vi "time_duration.vi"(8 "error in (no error)":errorcluster, 9 "out time":string[](array[string]), 10 "in time":string[](array[string]), 11 "Numeric":i32) -> (0 "error out":errorcluster, 1 "x+y 2":i32[](array[numeric]), 2 "time in second":dbl[](array[numeric]), 3 "x+y":i32[](array[numeric]))   [LabVIEW 2017]
panel:
  out "x+y 3":i32[](array[numeric])
  out "number 2":i32[](array[numeric])
  out "number":i32[](array[numeric])
  in  "Array 4":string[](array[string])
  out "Array 3":i32[](array[numeric])
  out "Array 2":i32[](array[numeric])
  out "Array":i32[](array[numeric])
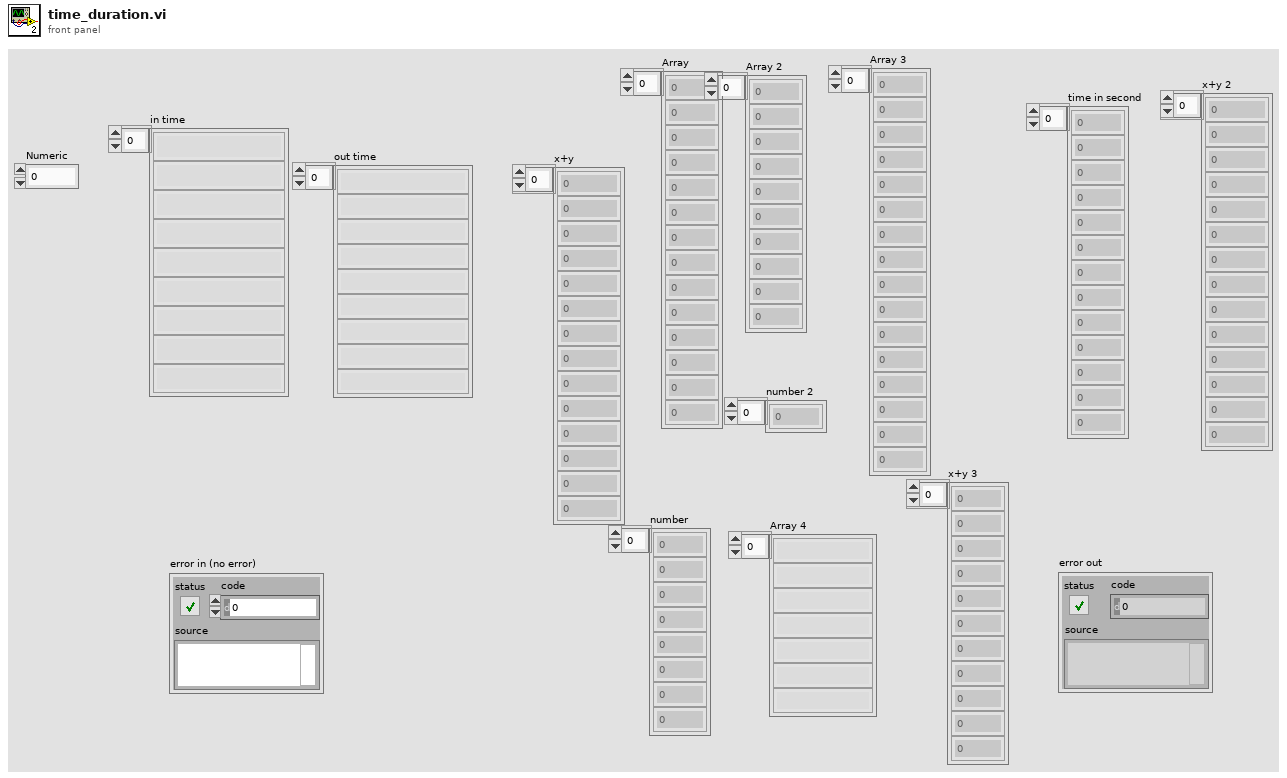
[diagram p1: front panel]
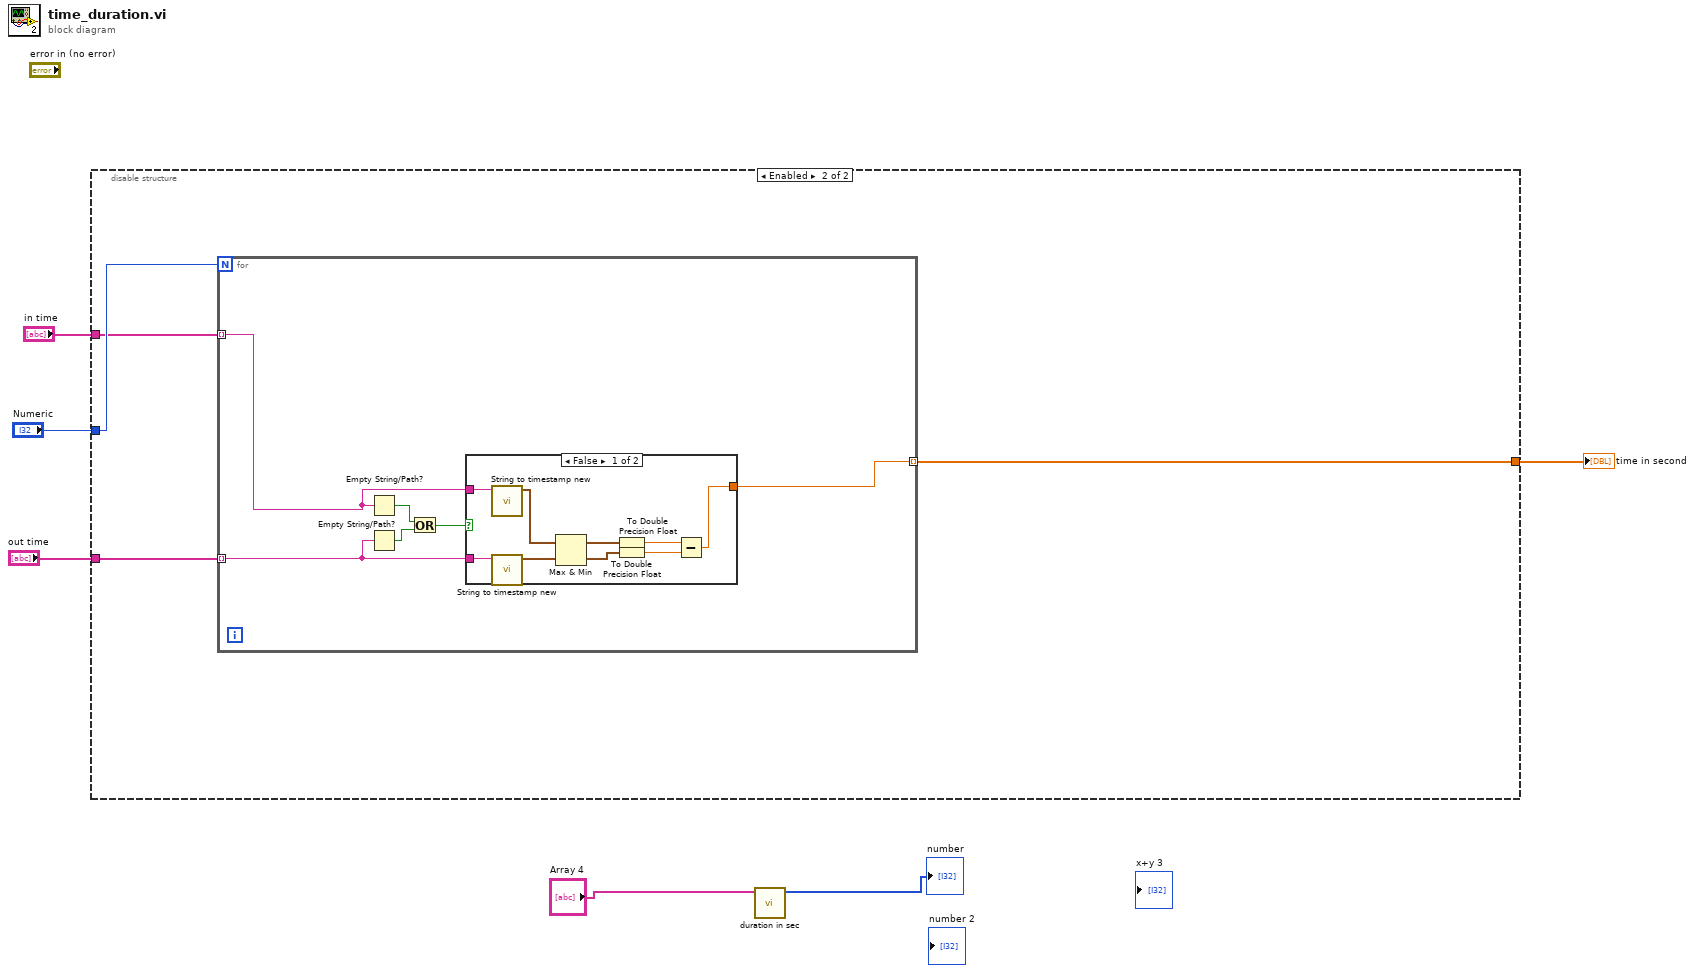
[diagram p0: block diagram]
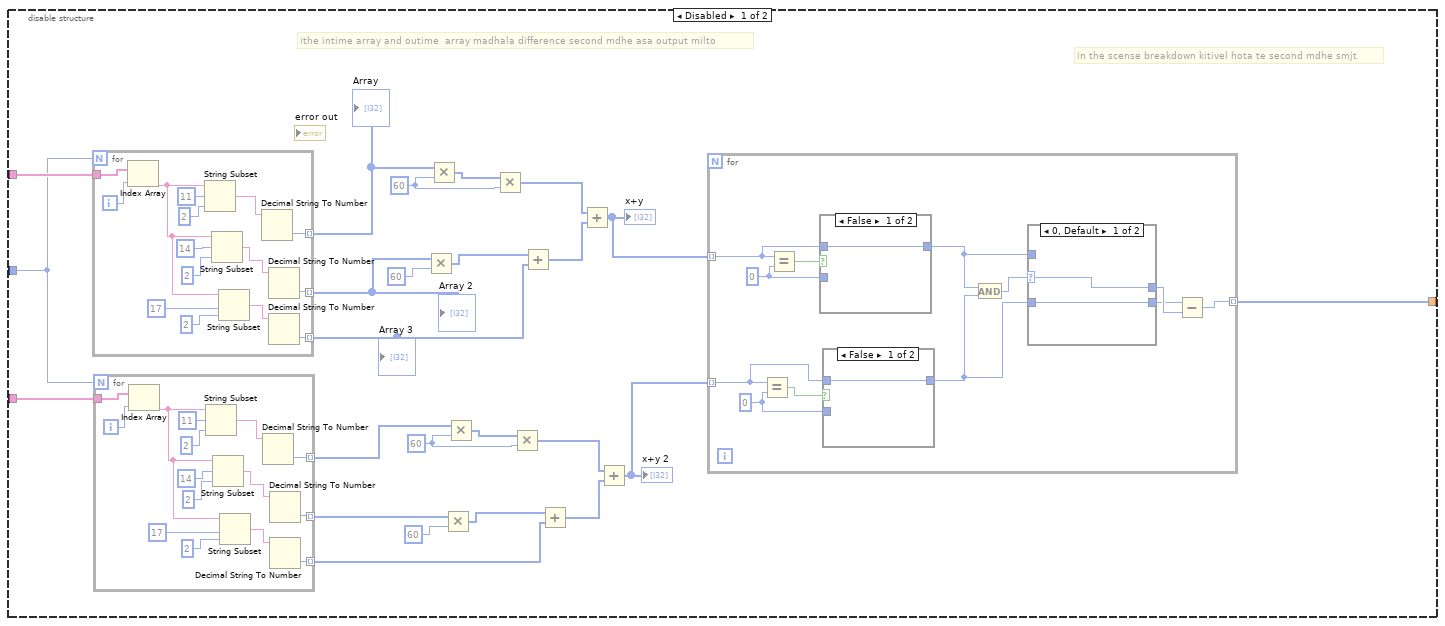
[diagram p2: hidden frame]
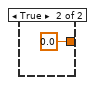
[diagram p6: hidden frame]
diagram:
  n1 = disable-structure shown="Enabled" {
    disable-tunnel: "in time" -> [w30 w83]
    disable-tunnel: "Numeric" -> [w29 w84]
    disable-tunnel: "out time" -> [w28 w82]
    disable-tunnel: [w7 w81] -> w3
    frame Disabled {
      w21 = 60
      w16 = 60
      # "in the scense breakdown kitivel hota te second mdhe smjt"
      # "ithe intime array and outime  array madhala difference second mdhe asa output milto"
      n2 = for {
        N: w29 -> [_]
        tunnel: w30 -> [w65]
        tunnel: [w53] -> w14 mode=indexing
        tunnel: [w52] -> w10 mode=indexing
        tunnel: [w51] -> w12 mode=indexing
        i -> [w63]
        n3 = Index Array(array=w65, index=w63) -> (element=w62:string)
        n4 = String Subset(string=w62, offset (0)=11, length (rest)=2 ("offset (0)")) -> (substring=w56:string)
        n5 = String Subset(string=w62, offset (0)=14, length (rest)=2 ("offset (0)")) -> (substring=w54:string)
        n6 = String Subset(string=w62, offset (0)=17, length (rest)=2 ("offset (0)")) -> (substring=w55:string)
        n7 = Decimal String To Number(string=w56) -> (number=w53:i32)  [unwired: 2 in, 1 out]
        n8 = Decimal String To Number(string=w54) -> (number=w52:i32)  [unwired: 2 in, 1 out]
        n9 = Decimal String To Number(string=w55) -> (number=w51:i32)  [unwired: 2 in, 1 out]
      }
      "Array" <- w14
      "Array 2" <- w10
      "Array 3" <- w12
      n10 = for {
        N: w29 -> [_]
        tunnel: w28 -> [w80]
        tunnel: [w68] -> w23 mode=indexing
        tunnel: [w67] -> w27 mode=indexing
        tunnel: [w66] -> w25 mode=indexing
        i -> [w78]
        n11 = Index Array(array=w80, index=w78) -> (element=w77:string)
        n12 = String Subset(string=w77, offset (0)=11, length (rest)=2 ("offset (0)")) -> (substring=w71:string)
        n13 = String Subset(string=w77, offset (0)=14, length (rest)=2 ("offset (0)")) -> (substring=w69:string)
        n14 = String Subset(string=w77, offset (0)=17, length (rest)=2 ("offset (0)")) -> (substring=w70:string)
        n15 = Decimal String To Number(string=w71) -> (number=w68:i32)  [unwired: 2 in, 1 out]
        n16 = Decimal String To Number(string=w69) -> (number=w67:i32)  [unwired: 2 in, 1 out]
        n17 = Decimal String To Number(string=w70) -> (number=w66:i32)  [unwired: 2 in, 1 out]
      }
      n18 = Multiply(x=w10, y=60) -> (x*y=w13:i32[])
      n19 = Multiply(x=w14, y=w16) -> (x*y=w15:i32[])
      n20 = Multiply(x=w27, y=60) -> (x*y=w24:i32[])
      n21 = Multiply(x=w23, y=w21) -> (x*y=w22:i32[])
      n22 = Multiply(x=w15, y=w16) -> (x*y=w18:i32[])
      n23 = Multiply(x=w22, y=w21) -> (x*y=w19:i32[])
      n24 = Add(x=w13, y=w12) -> (x+y=w17:i32[])
      n25 = Add(x=w24, y=w25) -> (x+y=w20:i32[])
      n26 = Add(x=w18, y=w17) -> (x+y=w9:i32[])
      "x+y" <- w9
      n27 = Add(x=w19, y=w20) -> (x+y=w8:i32[])
      "x+y 2" <- w8
      n28 = for {
        tunnel: w9 -> [w40] mode=indexing
        tunnel: w8 -> [w37] mode=indexing
        tunnel: [w31] -> w7 mode=indexing
        w38 = 0 ("y")
        w41 = 0 ("y")
        n29 = Equal?(x=w37, y=w38) -> (x = y?=w39:bool)
        n30 = Equal?(x=w40, y=w41) -> (x = y?=w42:bool)
        n31 = case shown="False" w42 {
          tunnel: [w49 w50] -> w32
          tunnel: w41 -> [_ w50]
          tunnel: w40 -> [w49 _]
          frame False {
          }
          frame True {
          }
        }
        n32 = case shown="False" w39 {
          tunnel: [w47 w48] -> w33
          tunnel: w38 -> [_ w48]
          tunnel: w37 -> [w47 _]
          frame False {
          }
          frame True {
          }
        }
        n33 = And(x=w32, y=w33) -> (x .and. y?=w36:i32)
        n34 = case shown="0, Default" w36 {
          selector: w36 -> [w44 _]
          tunnel: [w44 w45] -> w35
          tunnel: [w43 w46] -> w34
          tunnel: w33 -> [w43 w46]
          tunnel: w32 -> [_ w45]
          frame 0, Default {
          }
          frame 1.. {
          }
        }
        n35 = Subtract(x=w34, y=w35) -> (x-y=w31:i32)
      }
    }
    frame Enabled {
      n36 = for {
        N: w84 -> [_]
        tunnel: w83 -> [w86] mode=indexing
        tunnel: w82 -> [w87] mode=indexing
        tunnel: [w85] -> w81 mode=indexing
        n37 = Empty String/Path?(string/path=w86) -> (empty?=w89:bool)
        n38 = Empty String/Path?(string/path=w87) -> (empty?=w90:bool)
        n39 = Or(x=w89, y=w90) -> (x .or. y?=w88:bool)
        n40 = case shown="False" w88 {
          tunnel: [w93 0.0] -> w85
          tunnel: w86 -> [w92 _]
          tunnel: w87 -> [w91 _]
          frame False {
            n41 = call "String to timestamp new.vi"("String Timestamp"=w92) -> ("Timestamp"=w95:timestamp)  [unwired: 10 in]
            n42 = call "String to timestamp new.vi"("String Timestamp"=w91) -> ("Timestamp"=w94:timestamp)  [unwired: 10 in]
            n43 = Max & Min(x=w95, y=w94) -> (max(x,y)=w99:timestamp, min(x,y)=w98:timestamp)
            n44 = To Double Precision Float(number=w99) -> (double precision float=w97:dbl)
            n45 = To Double Precision Float(number=w98) -> (double precision float=w96:dbl)
            n46 = Subtract(x=w97, y=w96) -> (x-y=w93:dbl)
          }
          frame True {
          }
        }
      }
    }
  }
  "time in second" <- w3
  n47 = call "duration in sec.vi"("input time mm:ss"="Array 4") -> ("total in sec"=→"number":i32[])  [unwired: 10 in]
